vi "CAN参数设置.vi"() -> (10 "取消":bool, 12 "确定并启动":bool, 13 "工作方式 2":u8(ring) caption="工作方式" items=["Normal", "Listen Only"], 14 "CAN卡类型 2":u32(ring)=4 caption="CAN卡类型" items=["PCI5121"=1, "PCI9810"=2, "USBCAN1"=3, "USBCAN2"=4, "PCI9820"=5, "PCI5110"=7, "CANLite(mini)"=8, "ISA9620"=9, "ISA5420"=10, "PC104CAN"=11, "DNP9810"=13, "PCI9840B"=14, "PC104C2"=15, "PCI9820I"=16, "pec9920"=18, "USBCAN_E_U"=20, "USBCAN_2E_U"=21], 15 "设备索引号 2":u16(ring) caption="设备索引号" items=["0", "1", "2", "3", "4", "5", "6", "7", "8", "9", "10", "11", "12", "13", "14", "15", ""], 16 "波特率 2":T1(ring)=enum."500Kbps" caption="波特率", 17 "CAN端口 2":u16(ring) caption="CAN端口" items=["0", "1"], 18 "E-U_baud 2":u32(ring)=393223 caption="E-U_baud" items=["0x060003--1000Kbps"=393219, "0x060004--800Kbps"=393220, "0x060007--500Kbps"=393223, "0x1C0008--250Kbps"=1835016, "0x1C0011--125Kbps"=1835025, "0x160023--100Kbps"=1441827, "0x1C002C--50Kbps"=1835052, "0x1600B3--20Kbps"=1441971, "0x1C00E0--10Kbps"=1835232, "0x1C01C1--5Kbps"=1835457], 19 "滤波方式 2":u8(ring) caption="滤波方式" items=["Dual Filter", "Single Filter"])   [LabVIEW 2013]
panel:
  in  "确定并启动":bool
  in  "自适就CAN卡类型":bool=TRUE
  in  "退出":bool
  in  "确定":bool
  in  "E-U_baud":u32(ring)=1835016 caption="波特率" items=["500Kbps"=393223, "250Kbps"=1835016]
  in  "CAN卡类型":u32(ring)=21 items=["USBCAN1"=3, "USBCAN2"=4, "USBCAN_E_U"=20, "USBCAN_2E_U"=21]
  in  "工作方式":u8(ring) items=["一般模式", "只听模式"]
  in  "滤波方式":u8(ring) items=["双滤波方式", "单滤波方式"]
  in  "波特率":u16(ring)=9 items=["250Kbps", "500Kbps"]
  in  "CAN端口":u16(ring) items=["0", "1"]
  in  "设备索引号":u16(ring) items=["0", "1", "2", "3", "4", "5", "6", "7", "8", "9", "10", "11", "12", "13", "14", "15", ""]
  # "CAN参数配置"
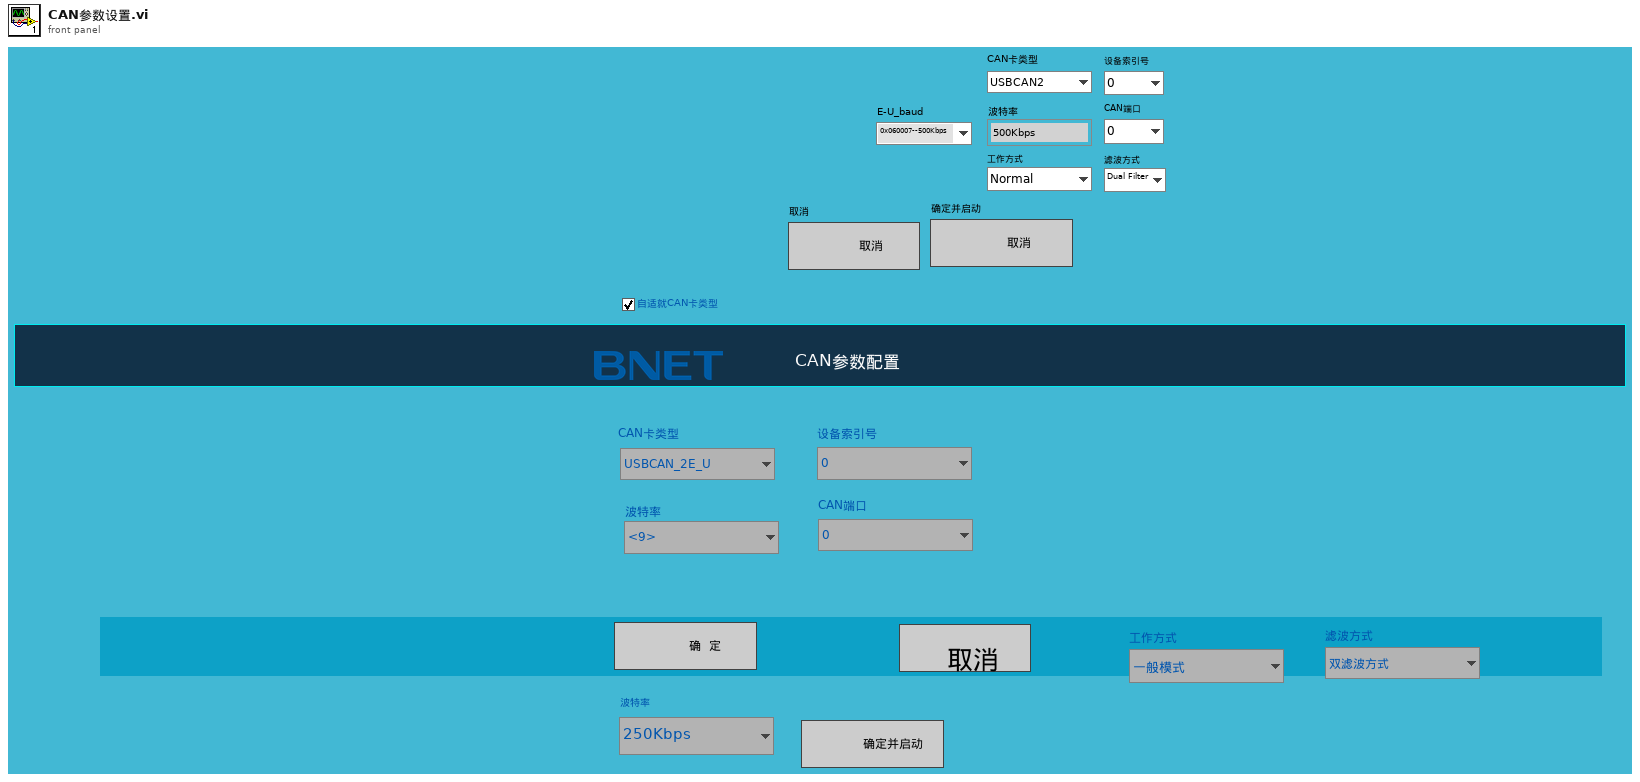
[diagram p1: front panel]
types:
  T1 = enum16{"5Kbps", "10Kbps", "20Kbps", "40Kbps", "50Kbps", "80Kbps", "100Kbps", "125Kbps", "200Kbps", "250Kbps", "400Kbps", "500Kbps", "666Kbps", "800Kbps", "1000Kbps"}
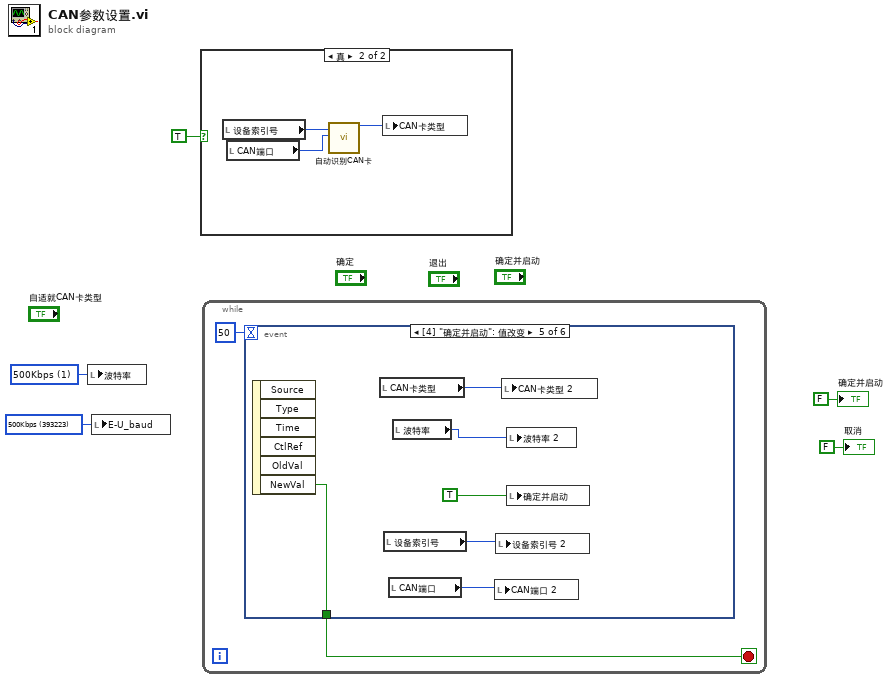
[diagram p0: block diagram]
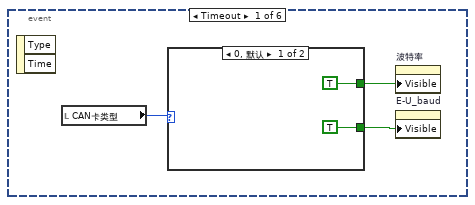
[diagram p3: hidden frame]
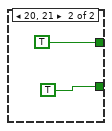
[diagram p4: hidden frame]
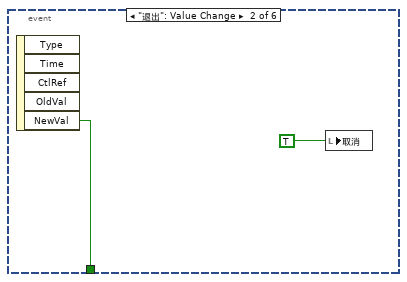
[diagram p5: hidden frame]
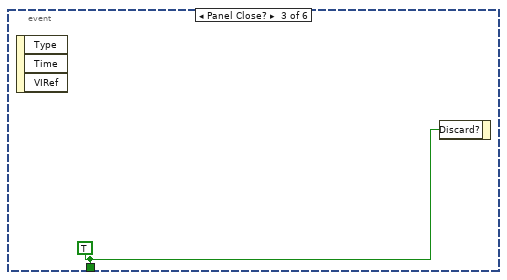
[diagram p6: hidden frame]
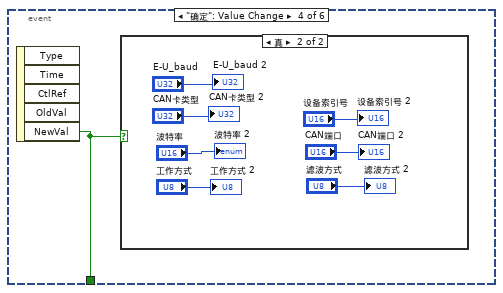
[diagram p7: hidden frame]
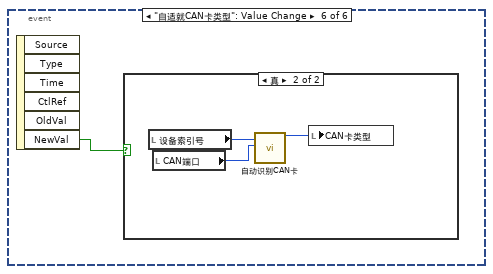
[diagram p9: hidden frame]
diagram:
  w4 = u32 393223 items=["500Kbps"=393223, "250Kbps"=1835016] ("E-U_baud")
  w5 = u16 1 items=["250Kbps", "500Kbps"] ("波特率")
  n1 = local write "波特率"(w5) -> ()
  n2 = local write "E-U_baud"(w4) -> ()
  n3 = case shown="真" TRUE {
    frame False {
    }
    frame True {
      n4 = local read "设备索引号"() -> (w7:u16)
      n5 = local read "CAN端口"() -> (w6:u16)
      n6 = call "自动识别CAN卡.vi"("设备索引号"=w7, "CAN端口"=w6) -> ("CAN卡类型 2"=w8:u32)  [unwired: 17 in]
      n7 = local write "CAN卡类型"(w8) -> ()
    }
  }
  n8 = while {
    stop <- w10 stop-if-true
    n9 = event shown="[4] \"确定并启动\": 值改变" {
      selector: _ -> [_ _ _ _ _ _]
      dyn-events: _ -> [_ _ _ _ _ _]
      timeout: 50 -> [_ _ _ _ _ _]
      tunnel: [_ w19 w20 w21 w33 _] -> w10
      event Timeout {
        n10 = event-data() -> ()  [unwired: 3 out]
        n11 = local read "CAN卡类型"() -> (w13:u32)
        n12 = case shown="0, 默认" w13 {
          tunnel: [TRUE TRUE] -> w12
          tunnel: [TRUE TRUE] -> w11
          frame 0, Default {
          }
          frame 20, 21 {
          }
        }
        n13 = property on="波特率" class="Ring (严格)"("Visible"=w12) -> ()  [unwired: 2 in, 2 out]
        n14 = property on="E-U_baud" class="Ring (严格)"("Visible"=w11) -> ()  [unwired: 2 in, 2 out]
      }
      event "退出": Value Change {
        n15 = event-data() -> ("NewVal"=w19:bool)  [unwired: 5 out]
        n16 = local write "取消"(TRUE ("取消")) -> ()
      }
      event Panel Close? {
        w20 = TRUE ("NewVal")
        n17 = event-data() -> ()  [unwired: 4 out]
        n18 = event-data("Discard?"=w20) -> ()  [unwired: 1 in, 1 out]
      }
      event "确定": Value Change {
        n19 = event-data() -> ("NewVal"=w21:bool)  [unwired: 5 out]
        n20 = case shown="真" w21 {
          frame False {
          }
          frame True {
            "E-U_baud 2" <- "E-U_baud"
            "CAN卡类型 2" <- "CAN卡类型"
            "波特率 2" <- "波特率"
            "工作方式 2" <- "工作方式"
            "设备索引号 2" <- "设备索引号"
            "CAN端口 2" <- "CAN端口"
            "滤波方式 2" <- "滤波方式"
          }
        }
      }
      event "确定并启动": Value Change {
        n21 = event-data() -> ("NewVal"=w33:bool)  [unwired: 6 out]
        n22 = local read "CAN卡类型"() -> (w32:u32)
        n23 = local read "设备索引号"() -> (w30:u16)
        n24 = local read "CAN端口"() -> (w29:u16)
        n25 = local read "波特率"() -> (w31:u16)
        n26 = local write "CAN端口 2"(w29) -> ()
        n27 = local write "设备索引号 2"(w30) -> ()
        n28 = local write "CAN卡类型 2"(w32) -> ()
        n29 = local write "波特率 2"(w31) -> ()
        n30 = local write "确定并启动"(TRUE ("确定并启动")) -> ()
      }
      event "自适就CAN卡类型": Value Change {
        n31 = event-data() -> ("NewVal"=w35:bool)  [unwired: 6 out]
        n32 = case shown="真" w35 {
          frame False {
          }
          frame True {
            n33 = local read "设备索引号"() -> (w37:u16)
            n34 = local read "CAN端口"() -> (w38:u16)
            n35 = call "自动识别CAN卡.vi"("设备索引号"=w37, "CAN端口"=w38) -> ("CAN卡类型 2"=w36:u32)  [unwired: 17 in]
            n36 = local write "CAN卡类型"(w36) -> ()
          }
        }
      }
    }
  }
  "确定并启动" <- FALSE ("确定并启动")
  "取消" <- FALSE ("取消")
